vi "make 1D array X dx.vi"(10 "dx":dbl, 11 "X":dbl) -> (3 "Array":dbl[](array[numeric]))   [LabVIEW 2020]
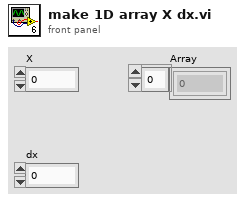
[diagram p1: front panel]
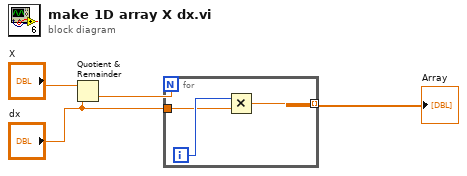
[diagram p0: block diagram]
diagram:
  n1 = Quotient & Remainder(x="X", y="dx") -> (floor(x/y)=w2:dbl)  [unwired: 1 out]
  n2 = for {
    N: w2 -> [_]
    tunnel: "dx" -> [w6]
    tunnel: [w5] -> w4 mode=indexing
    i -> [w7]
    n3 = Multiply(x=w7, y=w6) -> (x*y=w5:dbl)
  }
  "Array" <- w4
